vi "RecvMIMICCommand.vi"(0 "VISA resource name":refnum<visa-resource-name>="COM1", 1 "error in (no error)":errorcluster {"code" format="%.0x"}) -> (2 "Responce":string, 3 "return count":u32, 4 "error out":errorcluster)   [LabVIEW 2014]
panel:
  out "unsigned byte array":u8[](array[numeric]) format="%x"
  out "bytes read":u32
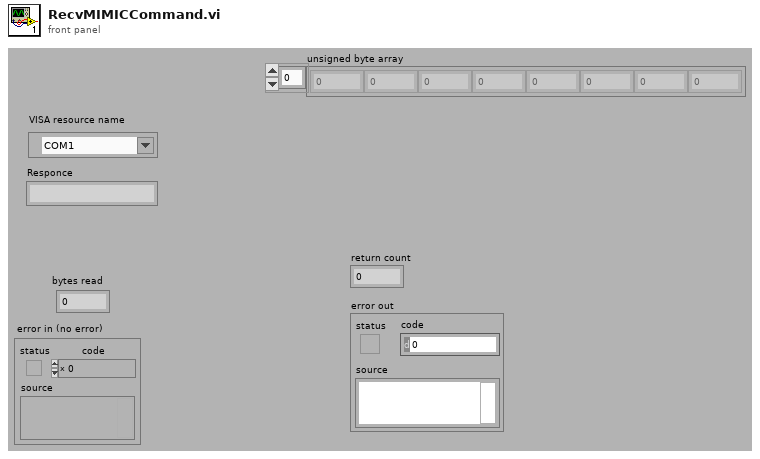
[diagram p1: front panel]
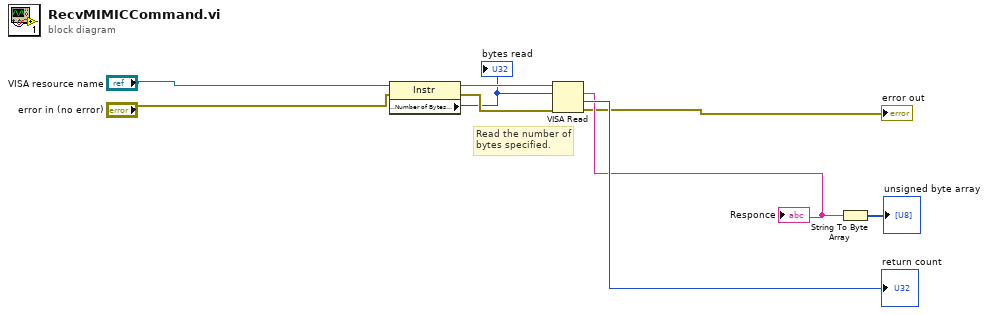
[diagram p0: block diagram]
diagram:
  # "Read the number of bytes specified."
  n1 = property class="Instr"(reference="VISA resource name", error in="error in (no error)") -> (reference out=w9:refnum<visa-resource-name>, error out=w8:errorcluster, "Serial Settings:Number of Bytes at Serial Port"=w4:u32)
  "bytes read" <- w4
  n2 = VISA Read(VISA resource name=w9, byte count=w4, error in (no error)=w8) -> (read buffer=w6:string, return count=→"return count":u32, error out=→"error out":errorcluster)  [unwired: 1 out]
  "Responce" <- w6
  n3 = String To Byte Array(string=w6) -> (unsigned byte array=→"unsigned byte array":u8[])
